vi "test_PhotonPoseEstimator_All.vi"(8 "error in (no error)":errorcluster) -> (0 "error out":errorcluster, 3 "Test Passed":bool)   [LabVIEW 2019]
panel:
  out "pnp dist trig solve":bool
  out "Avg Best":bool
  out "closest to last pose":bool
  out "closest to ref pose":bool
  out "closest to camera":bool
  out "lowest Ambiguity":bool
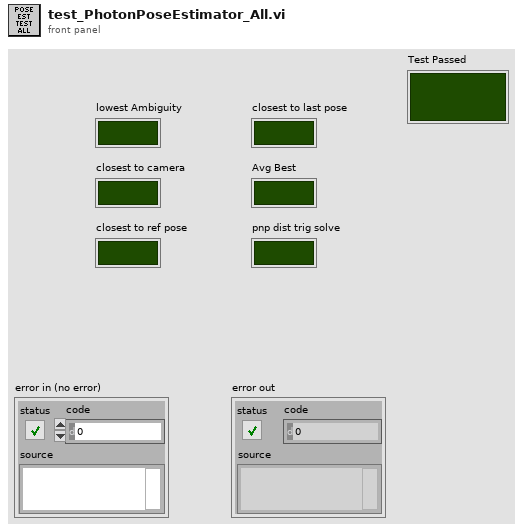
[diagram p1: front panel]
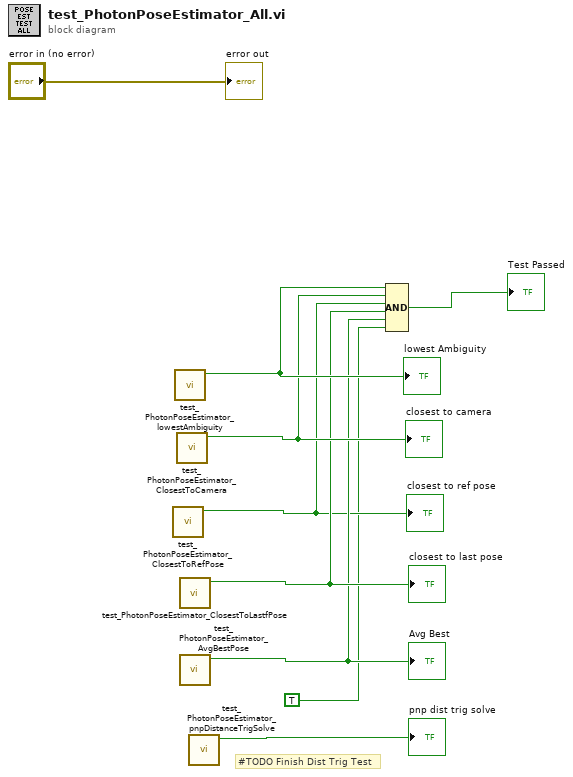
[diagram p0: block diagram]
diagram:
  # "#TODO Finish Dist Trig Test"
  n1 = call "test_PhotonPoseEstimator_ClosestToRefPose.vi"() -> ("Test Passed"=w3:bool)  [unwired: 10 in, 1 out]
  "closest to ref pose" <- w3
  n2 = call "test_PhotonPoseEstimator_lowestAmbiguity.vi"() -> ("Test Passed"=w7:bool)  [unwired: 10 in, 1 out]
  "lowest Ambiguity" <- w7
  n3 = call "test_PhotonPoseEstimator_ClosestToCamera.vi"() -> ("Test Passed"=w6:bool)  [unwired: 10 in, 1 out]
  "closest to camera" <- w6
  n4 = call "test_PhotonPoseEstimator_ClosestToLastfPose.vi"() -> ("Test Passed"=w5:bool)  [unwired: 10 in, 1 out]
  "closest to last pose" <- w5
  n5 = call "test_PhotonPoseEstimator_AvgBestPose.vi"() -> ("Test Passed"=w4:bool)  [unwired: 10 in, 1 out]
  "Avg Best" <- w4
  n6 = call "test_PhotonPoseEstimator_pnpDistanceTrigSolve.vi"() -> ("Test Passed"=→"pnp dist trig solve":bool)  [unwired: 10 in, 1 out]
  n7 = Compound Arithmetic op=AND(w7, w6, w3, w5, w4, TRUE) -> (→"Test Passed":bool)
  "error out" <- "error in (no error)"
